vi "PathChoose.vi"(6 "csv Name":string, 11 "?":T1) -> (3 "Path_Out":path)   [LabVIEW 2017]
uses:
  Ctrls/PathChoose.ctl
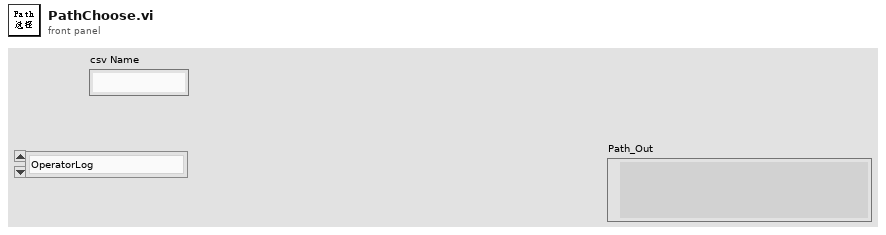
[diagram p1: front panel]
types:
  T1 = typedef "PathChoose.ctl" = enum16{"OperatorLog", "AutoRunLog", "AlmLog", "TestData", "AllTestData", "backup_nvm", "backup_before_flashing"}
  T2 = typedef "TesterInfo.ctl" = cluster{"Station Name":string, "Station Code":string, "ES NO.":string, "Tester ID":string, "PassMark Revision":string, "Rig ID":string, "Deamon_vision":string, "Project Name":string, "FFTesterPath":path, "Enable_User":bool, "Mode":enum16{"682"}, "MES":bool}
  T3 = typedef "HD Config.ctl" = cluster{" PC":cluster{"PC Address":u8[], "PC Port":i32}, "FCO":cluster{"COM":refnum<visa-resource-name>, "Baudrate":u32}, "DC Power ":cluster{"COM":refnum<visa-resource-name>, "Baudrate":u32}, "PW3336":cluster{"COM":refnum<visa-resource-name>, "Baudrate":u32}, "Lefoo":cluster{"COM":refnum<visa-resource-name>, "Baudrate":u32}, "Tempt&Hum":cluster{"COM":refnum<visa-resource-name>, "Baudrate":u32}, "DIPC":cluster{"COM":refnum<visa-resource-name>}, "Daemon":cluster{"IP Address":string, "Port":u16, "Retry":u16}, "URAT":cluster{"COM":refnum<visa-resource-name>, "Baudrate":u32}, "Fail_resume_mode":bool, "GRR":bool}
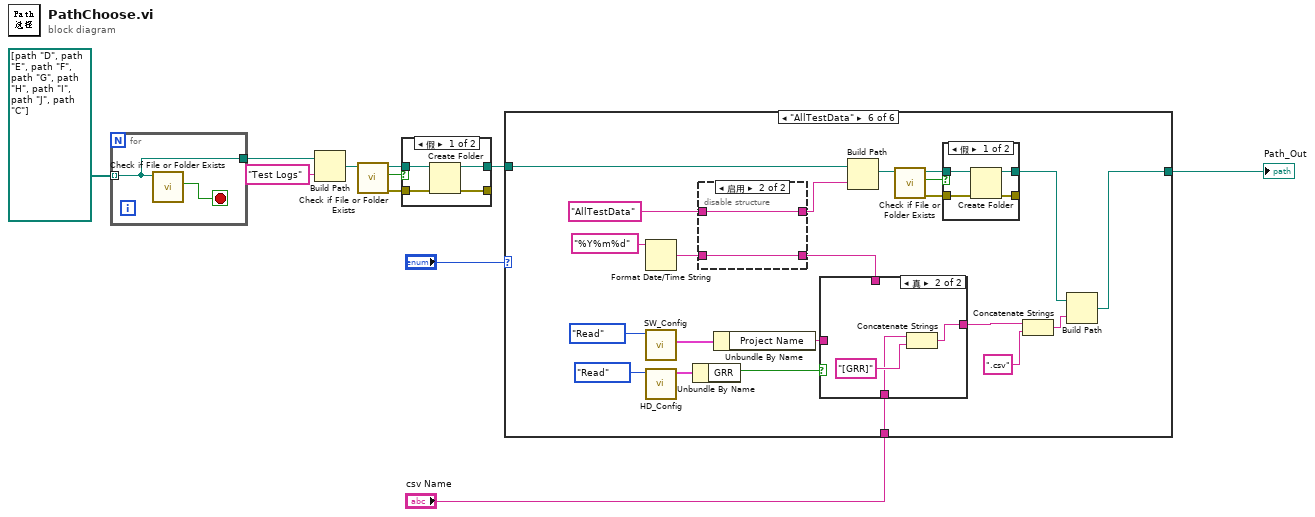
[diagram p0: block diagram]
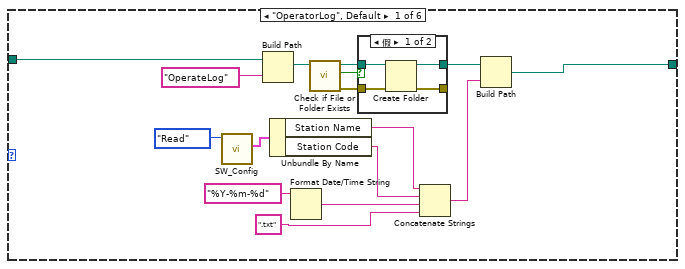
[diagram p2: hidden frame]
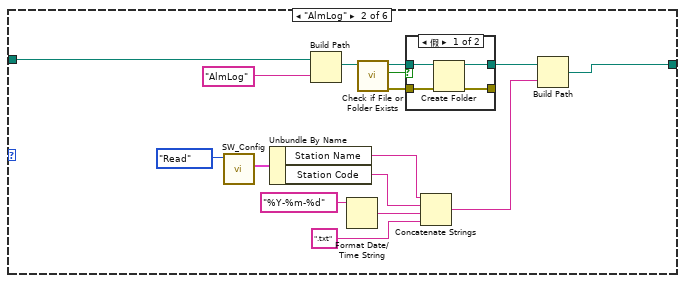
[diagram p4: hidden frame]
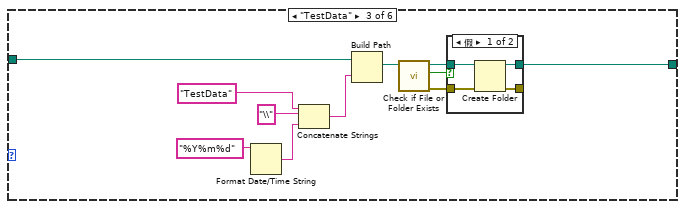
[diagram p6: hidden frame]
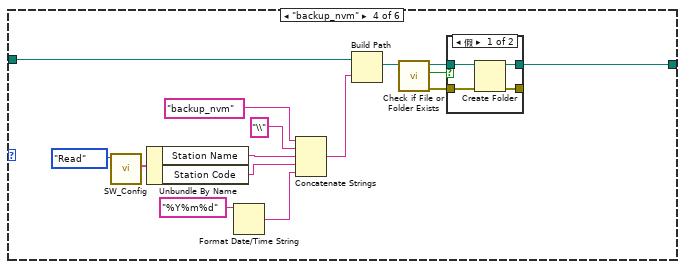
[diagram p8: hidden frame]
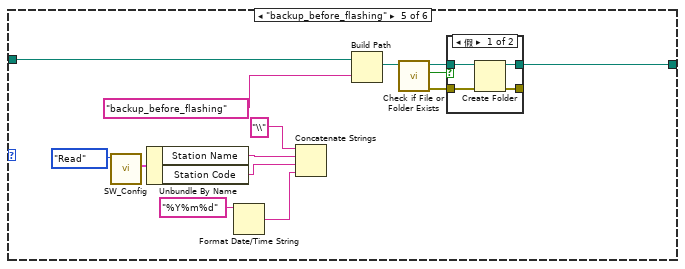
[diagram p10: hidden frame]
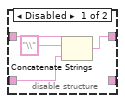
[diagram p13: hidden frame]
diagram:
  n1 = for {
    tunnel: path[] [path "D:/", path "E:/", path "F:/", path "G:/", path "H:/", path "I:/", path "J:/", path "C:/"] -> [w12] mode=indexing
    tunnel: [w12] -> w5
    stop <- w13 stop-if-true
    n2 = call <vilib>:"Check if File or Folder Exists.vi"("path"=w12) -> ("file or folder exists?"=w13:bool)  [unwired: 8 in, 2 out]
  }
  n3 = Build Path(base path=w5, name or relative path="Test Logs") -> (appended path=w3:path)
  n4 = call <vilib>:"Check if File or Folder Exists.vi"("path"=w3) -> ("error out"=w10:errorcluster, "file or folder exists?"=w11:bool, "dup path"=w9:path)  [unwired: 8 in]
  n5 = case shown="假" w11 {
    tunnel: w10 -> [w16 w18]
    tunnel: w9 -> [w17 w19]
    tunnel: [w14 w19] -> w8
    tunnel: [w15 w18] -> _
    frame False {
      n6 = Create Folder(path (use dialog)=w17, error in=w16) -> (created path=w14:path, error out=w15:errorcluster)  [unwired: 1 in, 1 out]
    }
    frame True {
    }
  }
  n7 = case shown="\"AllTestData\"" "?" {
    tunnel: w8 -> [w35 w57 w74 w95 w115 w143]
    tunnel: [w34 w56 w69 w90 w110 w129] -> w2
    tunnel: "csv Name" -> [_ _ _ _ _ w126]
    frame "OperatorLog", Default {
      n8 = call "SW_Config.vi"("Step"=enum16{"Initial", "Write", "Read"}."Read") -> ("SW Config out"=w20:T2)  [unwired: 9 in, 1 out]
      n9 = Build Path(base path=w35, name or relative path="OperateLog" ("OPfilename")) -> (appended path=w29:path)
      n10 = Unbundle By Name(w20) -> ("Station Name"=w26:string, "Station Code"=w25:string)
      n11 = Format Date/Time String(time format string (%c)="%Y-%m-%d" ("时间格式字符串(%c)")) -> (date/time string=w27:string)  [unwired: 2 in]
      n12 = call <vilib>:"Check if File or Folder Exists.vi"("path"=w29) -> ("error out"=w31:errorcluster, "file or folder exists?"=w30:bool, "dup path"=w32:path)  [unwired: 8 in]
      n13 = case shown="假" w30 {
        tunnel: w31 -> [w38 w40]
        tunnel: w32 -> [w39 w41]
        tunnel: [w36 w41] -> w28
        tunnel: [w37 w40] -> _
        frame False {
          n14 = Create Folder(path (use dialog)=w39, error in=w38) -> (created path=w36:path, error out=w37:errorcluster)  [unwired: 1 in, 1 out]
        }
        frame True {
        }
      }
      n15 = Concatenate Strings(w26, w25, w27, ".txt" ("字符串")) -> (w21:string)
      n16 = Build Path(base path=w28, name or relative path=w21) -> (appended path=w34:path)
    }
    frame "AlmLog" {
      n17 = call "SW_Config.vi"("Step"=enum16{"Initial", "Write", "Read"}."Read") -> ("SW Config out"=w42:T2)  [unwired: 9 in, 1 out]
      n18 = Unbundle By Name(w42) -> ("Station Name"=w44:string, "Station Code"=w43:string)
      n19 = Build Path(base path=w57, name or relative path="AlmLog" ("名称或相对路径")) -> (appended path=w51:path)
      n20 = Format Date/Time String(time format string (%c)="%Y-%m-%d" ("时间格式字符串(%c)")) -> (date/time string=w49:string)  [unwired: 2 in]
      n21 = call <vilib>:"Check if File or Folder Exists.vi"("path"=w51) -> ("error out"=w53:errorcluster, "file or folder exists?"=w52:bool, "dup path"=w54:path)  [unwired: 8 in]
      n22 = case shown="假" w52 {
        tunnel: w53 -> [w60 w62]
        tunnel: w54 -> [w61 w63]
        tunnel: [w58 w63] -> w47
        tunnel: [w59 w62] -> _
        frame False {
          n23 = Create Folder(path (use dialog)=w61, error in=w60) -> (created path=w58:path, error out=w59:errorcluster)  [unwired: 1 in, 1 out]
        }
        frame True {
        }
      }
      n24 = Concatenate Strings(w44, w43, w49, ".txt" ("字符串")) -> (w46:string)
      n25 = Build Path(base path=w47, name or relative path=w46) -> (appended path=w56:path)
    }
    frame "TestData" {
      n26 = Format Date/Time String(time format string (%c)="%Y%m%d") -> (date/time string=w68:string)  [unwired: 2 in]
      n27 = Concatenate Strings("TestData" ("名称或相对路径"), "\\" ("字符串"), w68) -> (w64:string)
      n28 = Build Path(base path=w74, name or relative path=w64) -> (appended path=w70:path)
      n29 = call <vilib>:"Check if File or Folder Exists.vi"("path"=w70) -> ("error out"=w72:errorcluster, "file or folder exists?"=w71:bool, "dup path"=w73:path)  [unwired: 8 in]
      n30 = case shown="假" w71 {
        tunnel: w72 -> [w77 w79]
        tunnel: w73 -> [w78 w80]
        tunnel: [w75 w80] -> w69
        tunnel: [w76 w79] -> _
        frame False {
          n31 = Create Folder(path (use dialog)=w78, error in=w77) -> (created path=w75:path, error out=w76:errorcluster)  [unwired: 1 in, 1 out]
        }
        frame True {
        }
      }
    }
    frame "backup_nvm" {
      n32 = call "SW_Config.vi"("Step"=enum16{"Initial", "Write", "Read"}."Read") -> ("SW Config out"=w85:T2)  [unwired: 9 in, 1 out]
      n33 = Unbundle By Name(w85) -> ("Station Name"=w83:string, "Station Code"=w82:string)
      n34 = Format Date/Time String(time format string (%c)="%Y%m%d") -> (date/time string=w81:string)  [unwired: 2 in]
      n35 = Concatenate Strings("backup_nvm" ("名称或相对路径"), "\\" ("字符串"), w83, w82, w81) -> (w86:string)
      n36 = Build Path(base path=w95, name or relative path=w86) -> (appended path=w91:path)
      n37 = call <vilib>:"Check if File or Folder Exists.vi"("path"=w91) -> ("error out"=w93:errorcluster, "file or folder exists?"=w92:bool, "dup path"=w94:path)  [unwired: 8 in]
      n38 = case shown="假" w92 {
        tunnel: w93 -> [w98 w100]
        tunnel: w94 -> [w99 w101]
        tunnel: [w96 w101] -> w90
        tunnel: [w97 w100] -> _
        frame False {
          n39 = Create Folder(path (use dialog)=w99, error in=w98) -> (created path=w96:path, error out=w97:errorcluster)  [unwired: 1 in, 1 out]
        }
        frame True {
        }
      }
    }
    frame "backup_before_flashing" {
      n40 = call "SW_Config.vi"("Step"=enum16{"Initial", "Write", "Read"}."Read") -> ("SW Config out"=w107:T2)  [unwired: 9 in, 1 out]
      n41 = Unbundle By Name(w107) -> ("Station Name"=w105:string, "Station Code"=w104:string)
      n42 = Format Date/Time String(time format string (%c)="%Y%m%d") -> (date/time string=w103:string)  [unwired: 2 in]
      n43 = Concatenate Strings("\\" ("字符串"), w105, w104, w103) -> ()  [unwired: 1 out]
      n44 = Build Path(base path=w115, name or relative path="backup_before_flashing" ("名称或相对路径")) -> (appended path=w111:path)
      n45 = call <vilib>:"Check if File or Folder Exists.vi"("path"=w111) -> ("error out"=w113:errorcluster, "file or folder exists?"=w112:bool, "dup path"=w114:path)  [unwired: 8 in]
      n46 = case shown="假" w112 {
        tunnel: w113 -> [w118 w120]
        tunnel: w114 -> [w119 w121]
        tunnel: [w116 w121] -> w110
        tunnel: [w117 w120] -> _
        frame False {
          n47 = Create Folder(path (use dialog)=w119, error in=w118) -> (created path=w116:path, error out=w117:errorcluster)  [unwired: 1 in, 1 out]
        }
        frame True {
        }
      }
    }
    frame "AllTestData" {
      n48 = Format Date/Time String(time format string (%c)="%Y%m%d") -> (date/time string=w136:string)  [unwired: 2 in]
      n49 = call "SW_Config.vi"("Step"=enum16{"Initial", "Write", "Read"}."Read") -> ("SW Config out"=w128:T2)  [unwired: 9 in, 1 out]
      n50 = call "HD_Config.vi"("Step"=enum16{"Initial", "Write", "Read"}."Read") -> ("HD Config out"=w123:T3)  [unwired: 9 in, 1 out]
      n51 = Unbundle By Name(w123) -> ("GRR"=w122:bool)
      n52 = disable-structure shown="启用" {
        disable-tunnel: "AllTestData" ("名称或相对路径") -> [w151 w153]
        disable-tunnel: w136 -> [w150 w152]
        disable-tunnel: [w148 w153] -> w135
        disable-tunnel: [_ w152] -> w127
        frame Disabled {
          n53 = Concatenate Strings(w151, "\\" ("字符串"), w150) -> (w148:string)
        }
        frame Enabled {
        }
      }
      n54 = Unbundle By Name(w128) -> ("Project Name"=w125:string)
      n55 = case shown="真" w122 {
        tunnel: [w144 w145] -> w133
        tunnel: w127 -> [_ _]
        tunnel: w126 -> [w144 w146]
        tunnel: w125 -> [_ _]
        frame False {
        }
        frame True {
          n56 = Concatenate Strings(w146, "[GRR]" ("字符串")) -> (w145:string)
        }
      }
      n57 = Build Path(base path=w143, name or relative path=w135) -> (appended path=w139:path)
      n58 = call <vilib>:"Check if File or Folder Exists.vi"("path"=w139) -> ("error out"=w141:errorcluster, "file or folder exists?"=w140:bool, "dup path"=w142:path)  [unwired: 8 in]
      n59 = case shown="假" w140 {
        tunnel: w141 -> [w156 w158]
        tunnel: w142 -> [w157 w159]
        tunnel: [w154 w159] -> w130
        tunnel: [w155 w158] -> _
        frame False {
          n60 = Create Folder(path (use dialog)=w157, error in=w156) -> (created path=w154:path, error out=w155:errorcluster)  [unwired: 1 in, 1 out]
        }
        frame True {
        }
      }
      n61 = Concatenate Strings(w133, ".csv" ("string")) -> (w134:string)
      n62 = Build Path(base path=w130, name or relative path=w134) -> (appended path=w129:path)
    }
  }
  "Path_Out" <- w2
